vi "RT_I2C Write.vi"(7 "Command (Write & Read)":u8(ring) items=["Write & Read", "Write", "Read"], 8 "error in":errorcluster, 9 "Number of Bytes to Write":u16, 10 "Data":u8[](array[numeric]), 11 "FPGA VI Reference In":T1) -> (0 "error out":errorcluster, 3 "FPGA VI Reference Out":T1)   [LabVIEW 2018]
uses:
  Data Def/RT_FPGA VI Reference.ctl
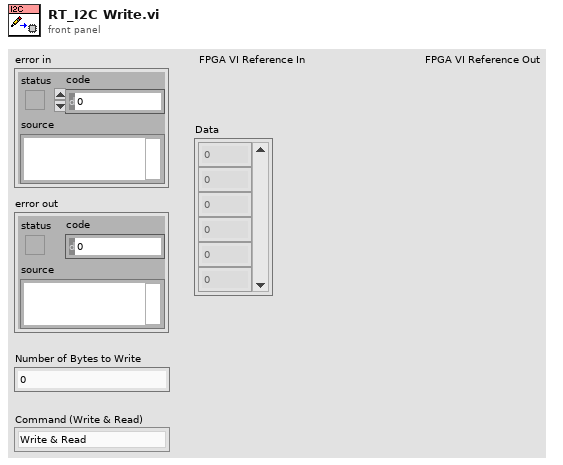
[diagram p1: front panel]
types:
  T1 = typedef "RT_FPGA VI Reference.ctl" = refnum<k20>
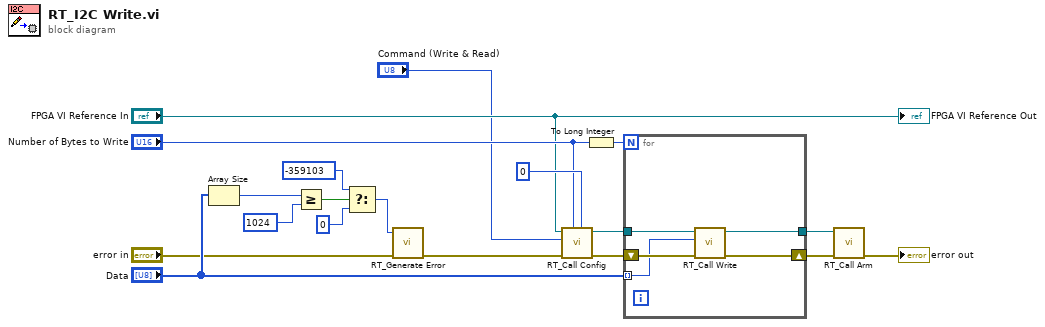
[diagram p0: block diagram]
diagram:
  n1 = Array Size(array="Data") -> (size(s)=w13:i32)
  n2 = Greater Or Equal?(x=w13, y=1024) -> (x >= y?=w16:bool)
  n3 = Select(t=-359103 ("Code"), s=w16, f=0 ("Code")) -> (s? t:f=w10:i32)
  n4 = call "RT_Generate Error.vi"("error in (no error)"="error in", "Code"=w10) -> ("error out"=w12:errorcluster)  [unwired: 9 in]
  n5 = call "RT_Call Config.vi"("Number of Bytes to Read"=u16 0, "Number of Bytes to Write"="Number of Bytes to Write", "error in"=w12, "Command (Write & Read)"="Command (Write & Read)", "FPGA VI Reference In"="FPGA VI Reference In") -> ("error out"=w5:errorcluster, "FPGA VI Reference Out"=w6:T1)  [unwired: 5 in]
  n6 = To Long Integer(number="Number of Bytes to Write") -> (32bit integer=w9:i32)
  n7 = for {
    N: w9 -> [_]
    tunnel: "Data" -> [w22] mode=indexing
    shift-right: [w23] -> w4
    shift-left: w5 -> [w24]
    tunnel: [w21] -> w3
    tunnel: w6 -> [w20]
    n8 = call "RT_Call Write.vi"("error in"=w24, "Data"=w22, "FPGA VI Reference In"=w20) -> ("error out"=w23:errorcluster, "FPGA VI Reference Out"=w21:T1)  [unwired: 7 in]
  }
  n9 = call "RT_Call Arm.vi"("error in"=w4, "FPGA VI Reference In"=w3) -> ("error out"=→"error out":errorcluster)  [unwired: 8 in, 1 out]
  "FPGA VI Reference Out" <- "FPGA VI Reference In"
